vi "Prepare Acquisition.vi"(8 "error in (no error)":errorcluster, 10 "Flash Settings":T1={"Exposure Time (ms)"=100.0, "Binning"=enum."2x2", "Scan Mode"=0, "Frames to Acquire"=1000.0, "Pixel Correction"=FALSE, "Frames to Skip"=0, "File Path"=path "", "Duty cycle"=0.0, "ALEX"=FALSE, "Shutter Enable"=[]} {"Exposure Time (ms)" min=1.0 max=10000.0 step=1.0}, 11 "Orca-Flash 4.0 in":refnum<class "Orca-Flash 4.0 V2.lvclass">) -> (0 "error out":errorcluster, 3 "Orca-Flash 4.0 out":refnum<class "Orca-Flash 4.0 V2.lvclass">)   [LabVIEW 2018, in "Orca-Flash 4.0 V2.lvlib" / "Orca-Flash 4.0 V2.lvclass"]
uses:
  Orca-Flash 4.0 V2.lvclass
  Resources/Type Defs/Camera Settings.ctl
  Orca-Flash 4.0 V2.lvclass/Orca-Flash 4.0 V2.ctl
  Resources/GLOBAL/GLOBAL Debug.vi
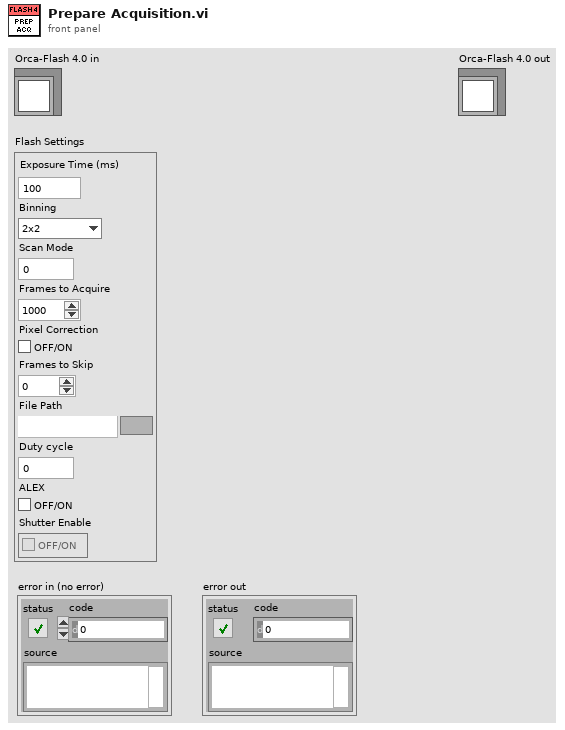
[diagram p1: front panel]
types:
  T1 = typedef "Camera Settings.ctl" = cluster{"Exposure Time (ms)":dbl, "Binning":enum16{"1x1", "2x2", "4x4"}, "Scan Mode":i32, "Frames to Acquire":dbl, "Pixel Correction":bool, "Frames to Skip":u32, "File Path":path, "Duty cycle":dbl, "ALEX":bool, "Shutter Enable":bool[]}
  T2 = cluster{"Horizontal Offset":i32, "Vertical Offset":i32, "Horizontal Size":i32, "Vertical Size":i32}
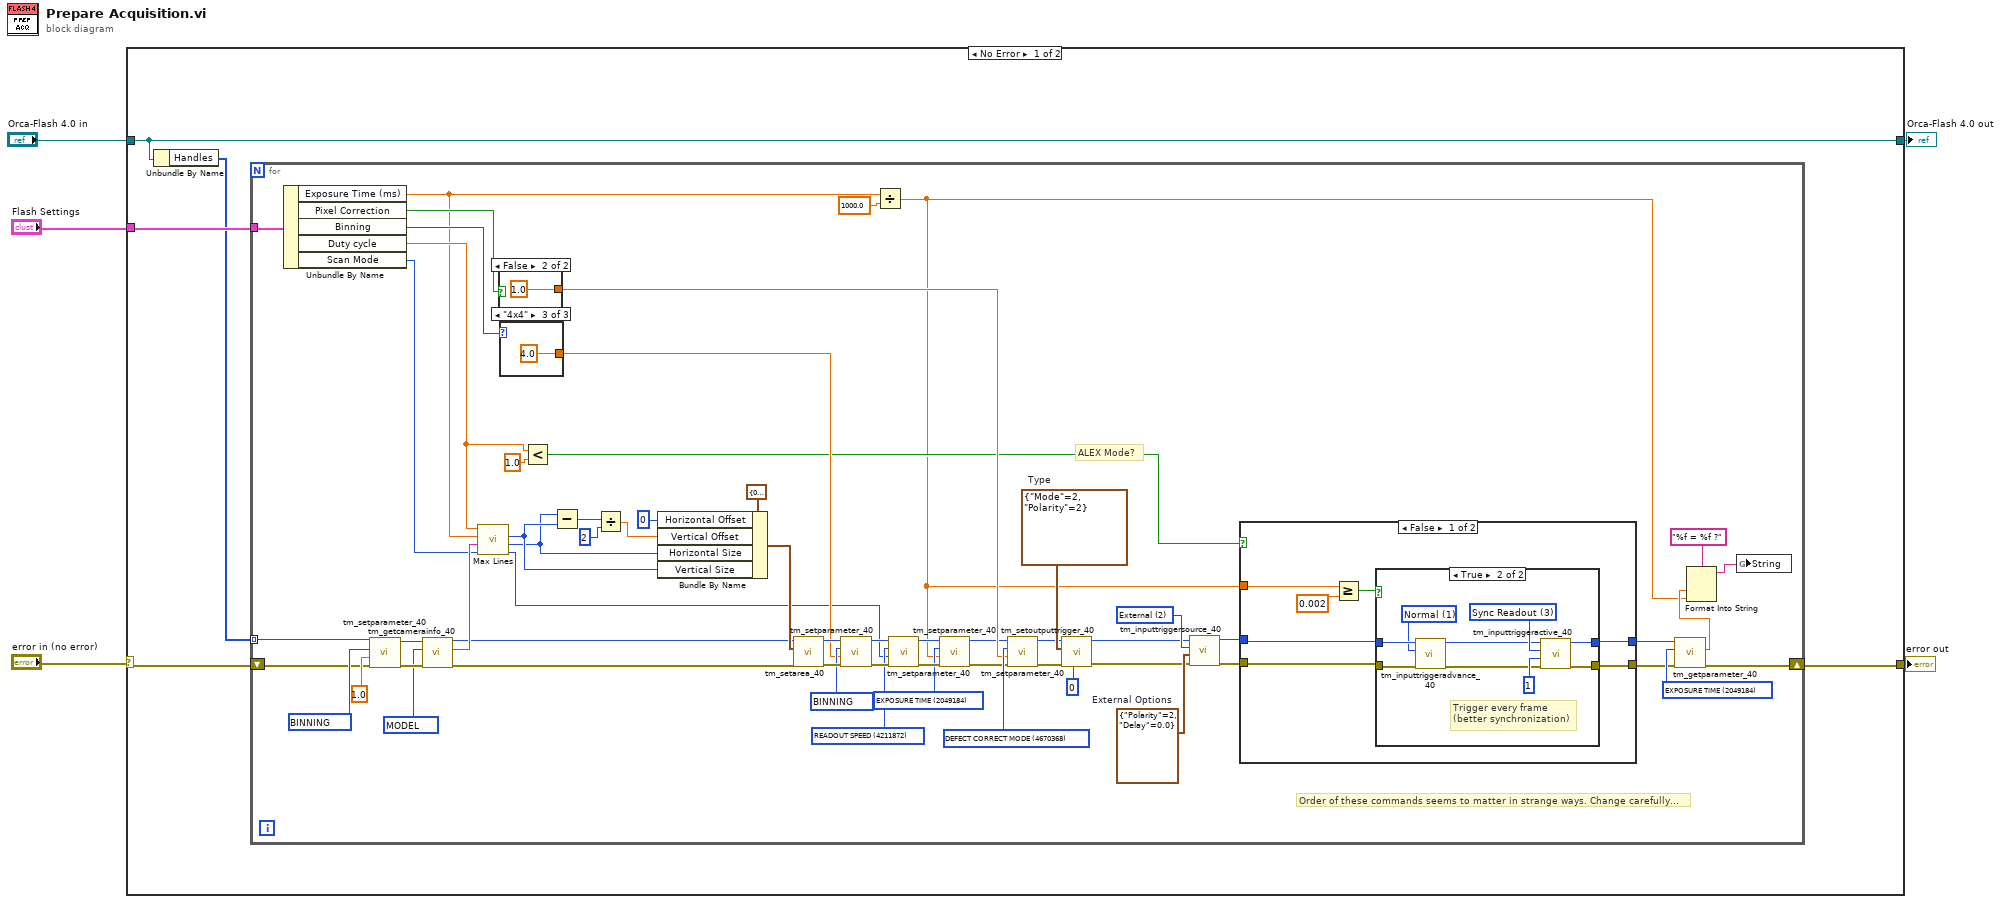
[diagram p0: block diagram]
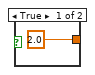
[diagram p2: hidden frame]
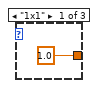
[diagram p3: hidden frame]
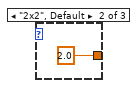
[diagram p4: hidden frame]
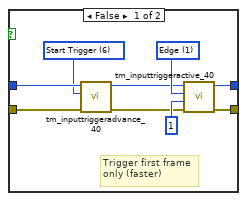
[diagram p5: hidden frame]
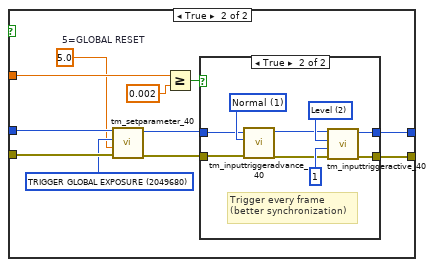
[diagram p6: hidden frame]
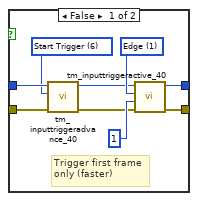
[diagram p7: hidden frame]
diagram:
  n1 = case shown="No Error" "error in (no error)" {
    selector: "error in (no error)" -> [w8 w131]
    tunnel: [w9 w131] -> w3
    tunnel: "Flash Settings" -> [w10 _]
    tunnel: "Orca-Flash 4.0 in" -> [w7 w130]
    tunnel: [w7 w130] -> w1
    frame No Error {
      n2 = Unbundle By Name(w7) -> ("Handles"=w6:u32[])
      n3 = for {
        tunnel: w10 -> [w70]
        shift-right: [w12] -> w9
        shift-left: w8 -> [w49]
        tunnel: w6 -> [w31] mode=indexing
        w18 = u32 2049184 items=["SENSOR MODE"=4212128, "READOUT SPEED"=4211872, "READOUT DIRECTION"=4211904, "BIT PER CHANNEL"=4342976, "TRIGGER GLOBAL EXPOSURE"=2049680, "TRIGGER DELAY"=1066480, "SYNC READOUT SYSTEM BLANK"=1066528, "SENSOR COOLER STATUS"=2115280, "EXPOSURE TIME"=2049184, "DEFECT CORRECT MODE"=4670368, "BINNING"=4215968, "TIMING READOUT TIME"=4223904, "INTERNAL FRAME RATE"=4225952, "INTERNAL FRAME INTERVAL"=4225968, "INTERNAL LINE SPEED"=4226000, "INTERNAL LINE INTERVAL"=4226016, "IMAGE WIDTH"=4343200, "IMAGE HEIGHT"=4343216, "IMAGE ROWBYTES"=4343232, "IMAGE FRAMEBYTES"=4343248, "IMAGE PIXEL TYPE"=4343296, "NUMBER OF OUTPUT TRIGGER CONNECTOR"=1852320, "OUTPUT TRIGGER SOURCE[0]"=1852576, "OUTPUT TRIGGER SOURCE[1]"=1852832, "OUTPUT TRIGGER SOURCE[2]"=1853088, "OUTPUT TRIGGER POLARITY[0]"=1852592, "OUTPUT TRIGGER POLARITY[1]"=1852848, "OUTPUT TRIGGER POLARITY[2]"=1853104, "OUTPUT TRIGGER ACTIVE[0]"=1852608, "OUTPUT TRIGGER ACTIVE[1]"=1852864, "OUTPUT TRIGGER ACTIVE[2]"=1853120, "OUTPUT TRIGGER DELAY[0]"=1852624, "OUTPUT TRIGGER DELAY[1]"=1852880, "OUTPUT TRIGGER DELAY[2]"=1853136, "OUTPUT TRIGGER PERIOD[0]"=1852640, "OUTPUT TRIGGER PERIOD[1]"=1852896, "OUTPUT TRIGGER PERIOD[2]"=1853152, "OUTPUT TRIGGER KIND[0]"=1852656, "OUTPUT TRIGGER KIND[1]"=1852912, "OUTPUT TRIGGER KIND[2]"=1853168, "OUTPUT TRIGGER PRE HSYNC COUNT"=1852704] ("Parameter")
        w29 = cluster{"Mode":u32, "Polarity":u32} {"Mode"=2, "Polarity"=2}  # Type
        w35 = 2 items=["Internal"=1, "External"=2, "Software"=3, "Master Pulse"=4] ("Source")
        w36 = cluster{"Polarity":i32, "Delay":dbl} {"Polarity"=2, "Delay"=0.0}  # External Options
        w42 = u32 67109124 items=["BUS"=67109121, "CAMERA ID"=67109122, "VENDOR"=67109123, "MODEL"=67109124, "CAMERA VERSION"=67109125, "DRIVER VERSION"=67109126, "MODULE VERSIOIN"=67109127, "DCAMAPI VERSION"=67109128] ("Info ID")
        w54 = u32 2049184 items=["SENSOR MODE"=4212128, "READOUT SPEED"=4211872, "READOUT DIRECTION"=4211904, "BIT PER CHANNEL"=4342976, "TRIGGER GLOBAL EXPOSURE"=2049680, "TRIGGER DELAY"=1066480, "SYNC READOUT SYSTEM BLANK"=1066528, "SENSOR COOLER STATUS"=2115280, "EXPOSURE TIME"=2049184, "DEFECT CORRECT MODE"=4670368, "BINNING"=4215968, "TIMING READOUT TIME"=4223904, "INTERNAL FRAME RATE"=4225952, "INTERNAL FRAME INTERVAL"=4225968, "INTERNAL LINE SPEED"=4226000, "INTERNAL LINE INTERVAL"=4226016, "IMAGE WIDTH"=4343200, "IMAGE HEIGHT"=4343216, "IMAGE ROWBYTES"=4343232, "IMAGE FRAMEBYTES"=4343248, "IMAGE PIXEL TYPE"=4343296, "NUMBER OF OUTPUT TRIGGER CONNECTOR"=1852320, "OUTPUT TRIGGER SOURCE[0]"=1852576, "OUTPUT TRIGGER SOURCE[1]"=1852832, "OUTPUT TRIGGER SOURCE[2]"=1853088, "OUTPUT TRIGGER POLARITY[0]"=1852592, "OUTPUT TRIGGER POLARITY[1]"=1852848, "OUTPUT TRIGGER POLARITY[2]"=1853104, "OUTPUT TRIGGER ACTIVE[0]"=1852608, "OUTPUT TRIGGER ACTIVE[1]"=1852864, "OUTPUT TRIGGER ACTIVE[2]"=1853120, "OUTPUT TRIGGER DELAY[0]"=1852624, "OUTPUT TRIGGER DELAY[1]"=1852880, "OUTPUT TRIGGER DELAY[2]"=1853136, "OUTPUT TRIGGER PERIOD[0]"=1852640, "OUTPUT TRIGGER PERIOD[1]"=1852896, "OUTPUT TRIGGER PERIOD[2]"=1853152, "OUTPUT TRIGGER KIND[0]"=1852656, "OUTPUT TRIGGER KIND[1]"=1852912, "OUTPUT TRIGGER KIND[2]"=1853168, "OUTPUT TRIGGER PRE HSYNC COUNT"=1852704] ("Parameter")
        w56 = u32 4670368 items=["SENSOR MODE"=4212128, "READOUT SPEED"=4211872, "READOUT DIRECTION"=4211904, "BIT PER CHANNEL"=4342976, "TRIGGER GLOBAL EXPOSURE"=2049680, "TRIGGER DELAY"=1066480, "SYNC READOUT SYSTEM BLANK"=1066528, "SENSOR COOLER STATUS"=2115280, "EXPOSURE TIME"=2049184, "DEFECT CORRECT MODE"=4670368, "BINNING"=4215968, "TIMING READOUT TIME"=4223904, "INTERNAL FRAME RATE"=4225952, "INTERNAL FRAME INTERVAL"=4225968, "INTERNAL LINE SPEED"=4226000, "INTERNAL LINE INTERVAL"=4226016, "IMAGE WIDTH"=4343200, "IMAGE HEIGHT"=4343216, "IMAGE ROWBYTES"=4343232, "IMAGE FRAMEBYTES"=4343248, "IMAGE PIXEL TYPE"=4343296, "NUMBER OF OUTPUT TRIGGER CONNECTOR"=1852320, "OUTPUT TRIGGER SOURCE[0]"=1852576, "OUTPUT TRIGGER SOURCE[1]"=1852832, "OUTPUT TRIGGER SOURCE[2]"=1853088, "OUTPUT TRIGGER POLARITY[0]"=1852592, "OUTPUT TRIGGER POLARITY[1]"=1852848, "OUTPUT TRIGGER POLARITY[2]"=1853104, "OUTPUT TRIGGER ACTIVE[0]"=1852608, "OUTPUT TRIGGER ACTIVE[1]"=1852864, "OUTPUT TRIGGER ACTIVE[2]"=1853120, "OUTPUT TRIGGER DELAY[0]"=1852624, "OUTPUT TRIGGER DELAY[1]"=1852880, "OUTPUT TRIGGER DELAY[2]"=1853136, "OUTPUT TRIGGER PERIOD[0]"=1852640, "OUTPUT TRIGGER PERIOD[1]"=1852896, "OUTPUT TRIGGER PERIOD[2]"=1853152, "OUTPUT TRIGGER KIND[0]"=1852656, "OUTPUT TRIGGER KIND[1]"=1852912, "OUTPUT TRIGGER KIND[2]"=1853168, "OUTPUT TRIGGER PRE HSYNC COUNT"=1852704] ("Parameter")
        w57 = u32 4211872 items=["SENSOR MODE"=4212128, "READOUT SPEED"=4211872, "READOUT DIRECTION"=4211904, "BIT PER CHANNEL"=4342976, "TRIGGER GLOBAL EXPOSURE"=2049680, "TRIGGER DELAY"=1066480, "SYNC READOUT SYSTEM BLANK"=1066528, "SENSOR COOLER STATUS"=2115280, "EXPOSURE TIME"=2049184, "DEFECT CORRECT MODE"=4670368, "BINNING"=4215968, "TIMING READOUT TIME"=4223904, "INTERNAL FRAME RATE"=4225952, "INTERNAL FRAME INTERVAL"=4225968, "INTERNAL LINE SPEED"=4226000, "INTERNAL LINE INTERVAL"=4226016, "IMAGE WIDTH"=4343200, "IMAGE HEIGHT"=4343216, "IMAGE ROWBYTES"=4343232, "IMAGE FRAMEBYTES"=4343248, "IMAGE PIXEL TYPE"=4343296, "NUMBER OF OUTPUT TRIGGER CONNECTOR"=1852320, "OUTPUT TRIGGER SOURCE[0]"=1852576, "OUTPUT TRIGGER SOURCE[1]"=1852832, "OUTPUT TRIGGER SOURCE[2]"=1853088, "OUTPUT TRIGGER POLARITY[0]"=1852592, "OUTPUT TRIGGER POLARITY[1]"=1852848, "OUTPUT TRIGGER POLARITY[2]"=1853104, "OUTPUT TRIGGER ACTIVE[0]"=1852608, "OUTPUT TRIGGER ACTIVE[1]"=1852864, "OUTPUT TRIGGER ACTIVE[2]"=1853120, "OUTPUT TRIGGER DELAY[0]"=1852624, "OUTPUT TRIGGER DELAY[1]"=1852880, "OUTPUT TRIGGER DELAY[2]"=1853136, "OUTPUT TRIGGER PERIOD[0]"=1852640, "OUTPUT TRIGGER PERIOD[1]"=1852896, "OUTPUT TRIGGER PERIOD[2]"=1853152, "OUTPUT TRIGGER KIND[0]"=1852656, "OUTPUT TRIGGER KIND[1]"=1852912, "OUTPUT TRIGGER KIND[2]"=1853168, "OUTPUT TRIGGER PRE HSYNC COUNT"=1852704] ("Parameter")
        w61 = u32 4215968 items=["SENSOR MODE"=4212128, "READOUT SPEED"=4211872, "READOUT DIRECTION"=4211904, "BIT PER CHANNEL"=4342976, "TRIGGER GLOBAL EXPOSURE"=2049680, "TRIGGER DELAY"=1066480, "SYNC READOUT SYSTEM BLANK"=1066528, "SENSOR COOLER STATUS"=2115280, "EXPOSURE TIME"=2049184, "DEFECT CORRECT MODE"=4670368, "BINNING"=4215968, "TIMING READOUT TIME"=4223904, "INTERNAL FRAME RATE"=4225952, "INTERNAL FRAME INTERVAL"=4225968, "INTERNAL LINE SPEED"=4226000, "INTERNAL LINE INTERVAL"=4226016, "IMAGE WIDTH"=4343200, "IMAGE HEIGHT"=4343216, "IMAGE ROWBYTES"=4343232, "IMAGE FRAMEBYTES"=4343248, "IMAGE PIXEL TYPE"=4343296, "NUMBER OF OUTPUT TRIGGER CONNECTOR"=1852320, "OUTPUT TRIGGER SOURCE[0]"=1852576, "OUTPUT TRIGGER SOURCE[1]"=1852832, "OUTPUT TRIGGER SOURCE[2]"=1853088, "OUTPUT TRIGGER POLARITY[0]"=1852592, "OUTPUT TRIGGER POLARITY[1]"=1852848, "OUTPUT TRIGGER POLARITY[2]"=1853104, "OUTPUT TRIGGER ACTIVE[0]"=1852608, "OUTPUT TRIGGER ACTIVE[1]"=1852864, "OUTPUT TRIGGER ACTIVE[2]"=1853120, "OUTPUT TRIGGER DELAY[0]"=1852624, "OUTPUT TRIGGER DELAY[1]"=1852880, "OUTPUT TRIGGER DELAY[2]"=1853136, "OUTPUT TRIGGER PERIOD[0]"=1852640, "OUTPUT TRIGGER PERIOD[1]"=1852896, "OUTPUT TRIGGER PERIOD[2]"=1853152, "OUTPUT TRIGGER KIND[0]"=1852656, "OUTPUT TRIGGER KIND[1]"=1852912, "OUTPUT TRIGGER KIND[2]"=1853168, "OUTPUT TRIGGER PRE HSYNC COUNT"=1852704] ("Parameter")
        w65 = u32 4215968 items=["SENSOR MODE"=4212128, "READOUT SPEED"=4211872, "READOUT DIRECTION"=4211904, "TRIGGER GLOBAL EXPOSURE"=2049680, "TRIGGER DELAY"=1066480, "INTERNAL TRIGGER HANDLING"=1066496, "SYNC READOUT SYSTEM BLANK"=1066528, "SENSOR TEMPERATURE"=2115232, "SENSOR COOLER STATUS"=2115280, "EXPOSURE TIME"=2049184, "DEFECT CORRECT MODE"=4670368, "BINNING"=4215968, "INTERNAL LINE SPEED"=4226000, "INTERNAL LINE INTERVAL"=4226016, "NUMBER OF OUTPUT TRIGGER CONNECTOR"=1852320, "OUTPUT TRIGGER SOURCE[0]"=1852576, "OUTPUT TRIGGER SOURCE[1]"=1852832, "OUTPUT TRIGGER SOURCE[2]"=1853088, "OUTPUT TRIGGER POLARITY[0]"=1852592, "OUTPUT TRIGGER POLARITY[1]"=1852848, "OUTPUT TRIGGER POLARITY[2]"=1853104, "OUTPUT TRIGGER ACTIVE[0]"=1852608, "OUTPUT TRIGGER ACTIVE[1]"=1852864, "OUTPUT TRIGGER ACTIVE[2]"=1853120, "OUTPUT TRIGGER DELAY[0]"=1852624, "OUTPUT TRIGGER DELAY[1]"=1852880, "OUTPUT TRIGGER DELAY[2]"=1853136, "OUTPUT TRIGGER PERIOD[0]"=1852640, "OUTPUT TRIGGER PERIOD[1]"=1852896, "OUTPUT TRIGGER PERIOD[2]"=1853152, "OUTPUT TRIGGER KIND[0]"=1852656, "OUTPUT TRIGGER KIND[1]"=1852912, "OUTPUT TRIGGER KIND[2]"=1853168, "OUTPUT TRIGGER BASE SENSOR[0]"=1852672, "OUTPUT TRIGGER BASE SENSOR[1]"=1852928, "OUTPUT TRIGGER BASE SENSOR[2]"=1853184, "OUTPUT TRIGGER PRE HSYNC COUNT"=1852704] ("Parameter")
        # "Order of these commands seems to matter in strange ways. Change carefully..."
        # "ALEX Mode?"
        n4 = Unbundle By Name(w70) -> ("Exposure Time (ms)"=w21:dbl, "Pixel Correction"=w40:bool, "Binning"=w39:enum16{"1x1", "2x2", "4x4"}, "Duty cycle"=w37:dbl, "Scan Mode"=w11:i32)
        n5 = call <userlib>:"tm_setparameter_40.vi"("error in (no error)"=w49, "Value in"=1.0, "Parameter"=w65, "Handle in"=w31) -> ("error out"=w45:errorcluster, "Handle out"=w46:u32)  [unwired: 6 in]
        n6 = call <userlib>:"tm_getcamerainfo_40.vi"("error in (no error)"=w45, "Info ID"=w42, "Handle in"=w46) -> ("error out"=w44:errorcluster, "String"=w43:string, "Handle out"=w41:u32)  [unwired: 6 in]
        n7 = call "Max Lines.vi"("scan mode in"=w11, "Camera Model"=w43, "Frame Time (ms)"=w21, "Duty cycle (fraction)"=w37) -> ("scan mode out"=w47:i32, "upper limit"=w48:i32, "Max Lines"=w53:i32)  [unwired: 3 in, 2 out]
        n8 = case shown="False" w40 {
          tunnel: [sgl 2.0 ("1 = OFF\n2 = ON") sgl 1.0 ("1 = OFF\n2 = ON")] -> w55
          frame True {
          }
          frame False {
          }
        }
        n9 = case shown="\"4x4\"" w39 {
          tunnel: [1.0 ("Value in") 2.0 ("Value in") 4.0 ("Value in")] -> w60
          frame "1x1" {
          }
          frame "2x2", Default {
          }
          frame "4x4" {
          }
        }
        n10 = Less?(x=w37, y=1.0) -> (x < y?=w32:bool)
        n11 = Subtract(x=w48, y=w53) -> (x-y=w52:i32)
        n12 = Divide(x=w52, y=2) -> (x/y=w50:dbl)
        n13 = Bundle By Name(cluster=T2 {"Horizontal Offset"=0, "Vertical Offset"=0, "Horizontal Size"=0, "Vertical Size"=0} ("Sub Region"), "Horizontal Offset"=0, "Vertical Offset"=w50, "Horizontal Size"=w48, "Vertical Size"=w53) -> (w67:T2)
        n14 = call <userlib>:"tm_setarea_40.vi"("error in (no error)"=w44, "Sub Region"=w67, "Handle in"=w41) -> ("error out"=w63:errorcluster, "Handle out"=w62:u32)  [unwired: 7 in]
        n15 = call <userlib>:"tm_setparameter_40.vi"("error in (no error)"=w63, "Value in"=w60, "Parameter"=w61, "Handle in"=w62) -> ("error out"=w58:errorcluster, "Handle out"=w59:u32)  [unwired: 6 in]
        n16 = Divide(x=w21, y=1000.0) -> (x/y=w17:dbl)
        n17 = call <userlib>:"tm_setparameter_40.vi"("error in (no error)"=w58, "Value in"=w47, "Parameter"=w57, "Handle in"=w59) -> ("error out"=w20:errorcluster, "Handle out"=w19:u32)  [unwired: 6 in]
        n18 = call <userlib>:"tm_setparameter_40.vi"("error in (no error)"=w20, "Value in"=w17, "Parameter"=w18, "Handle in"=w19) -> ("error out"=w13:errorcluster, "Handle out"=w14:u32)  [unwired: 6 in]
        n19 = call <userlib>:"tm_setparameter_40.vi"("error in (no error)"=w13, "Value in"=w55, "Parameter"=w56, "Handle in"=w14) -> ("error out"=w27:errorcluster, "Handle out"=w28:u32)  [unwired: 6 in]
        n20 = call <userlib>:"tm_setoutputtrigger_40.vi"("Port"=0, "error in (no error)"=w27, "Type"=w29, "Handle in"=w28) -> ("error out"=w25:errorcluster, "Handle out"=w26:u32)  [unwired: 6 in]
        n21 = call <userlib>:"tm_inputtriggersource_40.vi"("error in (no error)"=w25, "External Options"=w36, "Source"=w35, "Handle in"=w26) -> ("error out"=w33:errorcluster, "Handle out"=w34:u32)  [unwired: 6 in]
        n22 = case shown="False" w32 {
          tunnel: [w80 w111] -> w16
          tunnel: [w79 w110] -> w15
          tunnel: w17 -> [w76 w109]
          tunnel: w34 -> [w78 w108]
          tunnel: w33 -> [w77 w107]
          frame False {
            n23 = Greater Or Equal?(x=w76, y=0.002) -> (x >= y?=w82:bool)
            n24 = case shown="True" w82 {
              tunnel: [w84 w99] -> w80
              tunnel: [w83 w98] -> w79
              tunnel: w77 -> [w90 w96]
              tunnel: w78 -> [w91 w93]
              frame False {
                w87 = 1 items=["Edge"=1, "Level"=2, "Sync Readout"=3, "Point"=4] ("Active")
                w89 = 6 items=["Normal"=1, "PIV"=3, "Start Trigger"=6, "Multigate"=7, "Multiframe"=8] ("option")
                # "Trigger first frame\nonly (faster)"
                n25 = call <userlib>:"tm_inputtriggeradvance_40.vi"("error in (no error)"=w90, "option"=w89, "Handle in"=w91) -> ("error out"=w85:errorcluster, "Handle out"=w86:u32)  [unwired: 7 in]
                n26 = call <userlib>:"tm_inputtriggeractive_40.vi"("error in (no error)"=w85, "Times"=1, "Active"=w87, "Handle in"=w86) -> ("error out"=w83:errorcluster, "Handle out"=w84:u32)  [unwired: 6 in]
              }
              frame True {
                w92 = 1 items=["Normal"=1, "PIV"=3, "Start Trigger"=6, "Multigate"=7, "Multiframe"=8] ("option")
                w97 = 3 items=["Edge"=1, "Level"=2, "Sync Readout"=3, "Point"=4] ("Active")
                # "Trigger every frame\n(better synchronization)"
                n27 = call <userlib>:"tm_inputtriggeradvance_40.vi"("error in (no error)"=w96, "option"=w92, "Handle in"=w93) -> ("error out"=w95:errorcluster, "Handle out"=w94:u32)  [unwired: 7 in]
                n28 = call <userlib>:"tm_inputtriggeractive_40.vi"("error in (no error)"=w95, "Times"=1, "Active"=w97, "Handle in"=w94) -> ("error out"=w98:errorcluster, "Handle out"=w99:u32)  [unwired: 6 in]
              }
            }
          }
          frame True {
            w101 = 5.0  # 5=GLOBAL RESET
            w104 = u32 2049680 items=["SENSOR MODE"=4212128, "READOUT SPEED"=4211872, "READOUT DIRECTION"=4211904, "BIT PER CHANNEL"=4342976, "TRIGGER GLOBAL EXPOSURE"=2049680, "TRIGGER DELAY"=1066480, "SYNC READOUT SYSTEM BLANK"=1066528, "SENSOR COOLER STATUS"=2115280, "EXPOSURE TIME"=2049184, "DEFECT CORRECT MODE"=4670368, "BINNING"=4215968, "TIMING READOUT TIME"=4223904, "INTERNAL FRAME RATE"=4225952, "INTERNAL FRAME INTERVAL"=4225968, "INTERNAL LINE SPEED"=4226000, "INTERNAL LINE INTERVAL"=4226016, "IMAGE WIDTH"=4343200, "IMAGE HEIGHT"=4343216, "IMAGE ROWBYTES"=4343232, "IMAGE FRAMEBYTES"=4343248, "IMAGE PIXEL TYPE"=4343296, "NUMBER OF OUTPUT TRIGGER CONNECTOR"=1852320, "OUTPUT TRIGGER SOURCE[0]"=1852576, "OUTPUT TRIGGER SOURCE[1]"=1852832, "OUTPUT TRIGGER SOURCE[2]"=1853088, "OUTPUT TRIGGER POLARITY[0]"=1852592, "OUTPUT TRIGGER POLARITY[1]"=1852848, "OUTPUT TRIGGER POLARITY[2]"=1853104, "OUTPUT TRIGGER ACTIVE[0]"=1852608, "OUTPUT TRIGGER ACTIVE[1]"=1852864, "OUTPUT TRIGGER ACTIVE[2]"=1853120, "OUTPUT TRIGGER DELAY[0]"=1852624, "OUTPUT TRIGGER DELAY[1]"=1852880, "OUTPUT TRIGGER DELAY[2]"=1853136, "OUTPUT TRIGGER PERIOD[0]"=1852640, "OUTPUT TRIGGER PERIOD[1]"=1852896, "OUTPUT TRIGGER PERIOD[2]"=1853152, "OUTPUT TRIGGER KIND[0]"=1852656, "OUTPUT TRIGGER KIND[1]"=1852912, "OUTPUT TRIGGER KIND[2]"=1853168, "OUTPUT TRIGGER PRE HSYNC COUNT"=1852704] ("Parameter")
            n29 = call <userlib>:"tm_setparameter_40.vi"("error in (no error)"=w107, "Value in"=w101, "Parameter"=w104, "Handle in"=w108) -> ("error out"=w102:errorcluster, "Handle out"=w103:u32)  [unwired: 6 in]
            n30 = Greater Or Equal?(x=w109, y=0.002) -> (x >= y?=w105:bool)
            n31 = case shown="True" w105 {
              tunnel: [w114 w128] -> w111
              tunnel: [w115 w127] -> w110
              tunnel: w102 -> [w117 w121]
              tunnel: w103 -> [w118 w124]
              frame False {
                w112 = 6 items=["Normal"=1, "PIV"=3, "Start Trigger"=6, "Multigate"=7, "Multiframe"=8] ("option")
                w120 = 1 items=["Edge"=1, "Level"=2, "Sync Readout"=3, "Point"=4] ("Active")
                # "Trigger first frame\nonly (faster)"
                n32 = call <userlib>:"tm_inputtriggeradvance_40.vi"("error in (no error)"=w117, "option"=w112, "Handle in"=w118) -> ("error out"=w116:errorcluster, "Handle out"=w113:u32)  [unwired: 7 in]
                n33 = call <userlib>:"tm_inputtriggeractive_40.vi"("error in (no error)"=w116, "Times"=1, "Active"=w120, "Handle in"=w113) -> ("error out"=w115:errorcluster, "Handle out"=w114:u32)  [unwired: 6 in]
              }
              frame True {
                w125 = 1 items=["Normal"=1, "PIV"=3, "Start Trigger"=6, "Multigate"=7, "Multiframe"=8] ("option")
                w126 = 2 items=["Edge"=1, "Level"=2, "Sync Readout"=3, "Point"=4] ("Active")
                # "Trigger every frame\n(better synchronization)"
                n34 = call <userlib>:"tm_inputtriggeradvance_40.vi"("error in (no error)"=w121, "option"=w125, "Handle in"=w124) -> ("error out"=w122:errorcluster, "Handle out"=w123:u32)  [unwired: 7 in]
                n35 = call <userlib>:"tm_inputtriggeractive_40.vi"("error in (no error)"=w122, "Times"=1, "Active"=w126, "Handle in"=w123) -> ("error out"=w127:errorcluster, "Handle out"=w128:u32)  [unwired: 6 in]
              }
            }
          }
        }
        n36 = call <userlib>:"tm_getparameter_40.vi"("error in (no error)"=w15, "Parameter"=w54, "Handle in"=w16) -> ("error out"=w12:errorcluster, "Value out"=w22:dbl)  [unwired: 6 in, 1 out]
        n37 = Format Into String(format string="%f = %f ?", w22, w17) -> (resulting string=w24:string)  [unwired: 2 in, 1 out]
        n38 = global write "GLOBAL Debug.vi" "String"(w24) -> ()
      }
    }
    frame Error {
    }
  }
  "error out" <- w3
  "Orca-Flash 4.0 out" <- w1
